vi "Transfer Count (Framework).vi"(8 "error in (no error)":errorcluster, 11 "Framework Configuration in":T1) -> (0 "error out":errorcluster, 2 "transfer count":i32, 3 "Framework Configuration out":T1)   [LabVIEW 2017, in "DSF Core.lvlib"]
uses:
  DSF Core.lvlib
  Typedefs/DSF Engine Framework Configuration.ctl
  Typedefs/DSF Engine Plugin Configuration.ctl
  Typedefs/DSF Timing Info.ctl
  Typedefs/DSF Engine Plugin Thread Configuration.ctl
  Typedefs/DSF Settings Info.ctl
  Typedefs/DSF Engine Transfer Group Configuration.ctl
  Typedefs/DSF Direction.ctl
  Typedefs/DSF Engine Transfer Configuration.ctl
  Typedefs/DSF Byte Order.ctl
  Typedefs/DSF Engine Channel Configuration.ctl
  Typedefs/DSF Data Type.ctl
  Typedefs/DSF Timeout Behavior.ctl
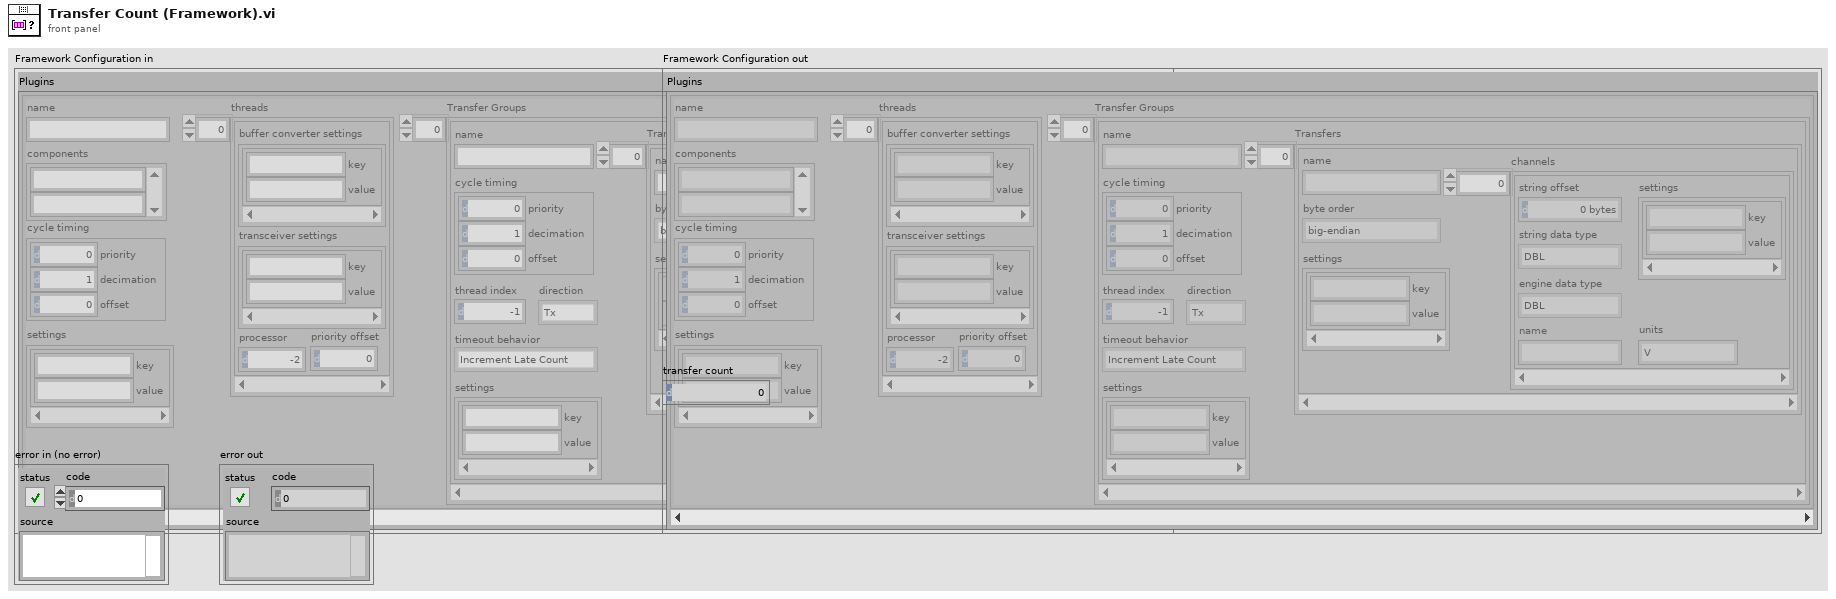
[diagram p1: front panel]
types:
  T1 = typedef "DSF Core.lvlib/DSF Engine Framework Configuration.ctl" = cluster{"Plugins":T2[]}
  T2 = typedef "DSF Core.lvlib/DSF Engine Plugin Configuration.ctl" = cluster{"name":string, "components":string[], "cycle timing":T3, "threads":T4[], "Transfer Groups":T6[], "settings":T5}
  T3 = typedef "DSF Core.lvlib/DSF Timing Info.ctl" = cluster{"priority":u64, "decimation":u64, "offset":u64}
  T4 = typedef "DSF Core.lvlib/DSF Engine Plugin Thread Configuration.ctl" = cluster{"buffer converter settings":T5, "transceiver settings":T5, "processor":i32, "priority offset":i16}
  T5 = typedef "DSF Core.lvlib/DSF Settings Info.ctl" = cluster{"key":string, "value":string}[]
  T6 = typedef "DSF Core.lvlib/DSF Engine Transfer Group Configuration.ctl" = cluster{"name":string, "direction":T7, "cycle timing":T3, "thread index":i32, "settings":T5, "Transfers":T8[], "timeout behavior":T12}
  T7 = typedef "DSF Core.lvlib/DSF Direction.ctl" = enum8{"Tx", "Rx"}
  T8 = typedef "DSF Core.lvlib/DSF Engine Transfer Configuration.ctl" = cluster{"name":string, "byte order":T9, "settings":T5, "channels":T10[]}
  T9 = typedef "DSF Core.lvlib/DSF Byte Order.ctl" = enum8{"big-endian", "little-endian"}
  T10 = typedef "DSF Core.lvlib/DSF Engine Channel Configuration.ctl" = cluster{"string offset":u64, "string data type":T11, "engine data type":T11, "name":string, "settings":T5, "units":string}
  T11 = typedef "DSF Core.lvlib/DSF Data Type.ctl" = enum8{"Bool", "SGL", "DBL", "I8", "I16", "I32", "I64", "U8", "U16", "U32", "U64"}
  T12 = typedef "DSF Core.lvlib/DSF Timeout Behavior.ctl" = enum8{"Increment Late Count", "Throw Error"}
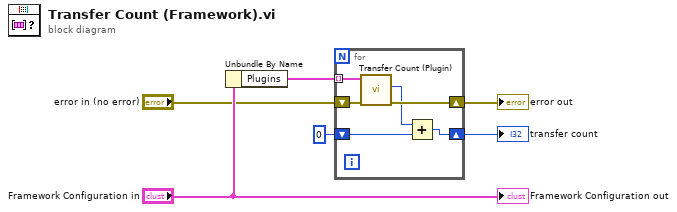
[diagram p0: block diagram]
diagram:
  n1 = Unbundle By Name("Framework Configuration in") -> ("Plugins"=w3:T2[])
  n2 = for {
    tunnel: w3 -> [w10] mode=indexing
    shift-right: [w12] -> w5
    shift-left: 0 -> [w11]
    shift-right: [w8] -> w1
    shift-left: "error in (no error)" -> [w9]
    n3 = call "Transfer Count (Plugin).vi"("error in (no error)"=w9, "Plugin Configuration in"=w10) -> ("error out"=w8:errorcluster, "transfer count"=w7:i32)  [unwired: 7 in, 1 out]
    n4 = Add(x=w7, y=w11) -> (x+y=w12:i32)
  }
  "transfer count" <- w5
  "error out" <- w1
  "Framework Configuration out" <- "Framework Configuration in"
